vi "Autonomous Independent.vi"   [LabVIEW 2020]
doc: "This VI is called when autonomous begins, and will automatically be terminated when autonomous ends. You can carry out timed or sensor driven robot movement independently without needing to return to the caller."
uses:
  <vilib>/Rock Robotics/Network Tables/NT Read String.vi
  Robot Global Data.vi
panel:
  # "Be sure to right-click and choose Data Operations>>Make Current Value default if you want to save the array values with the VI"
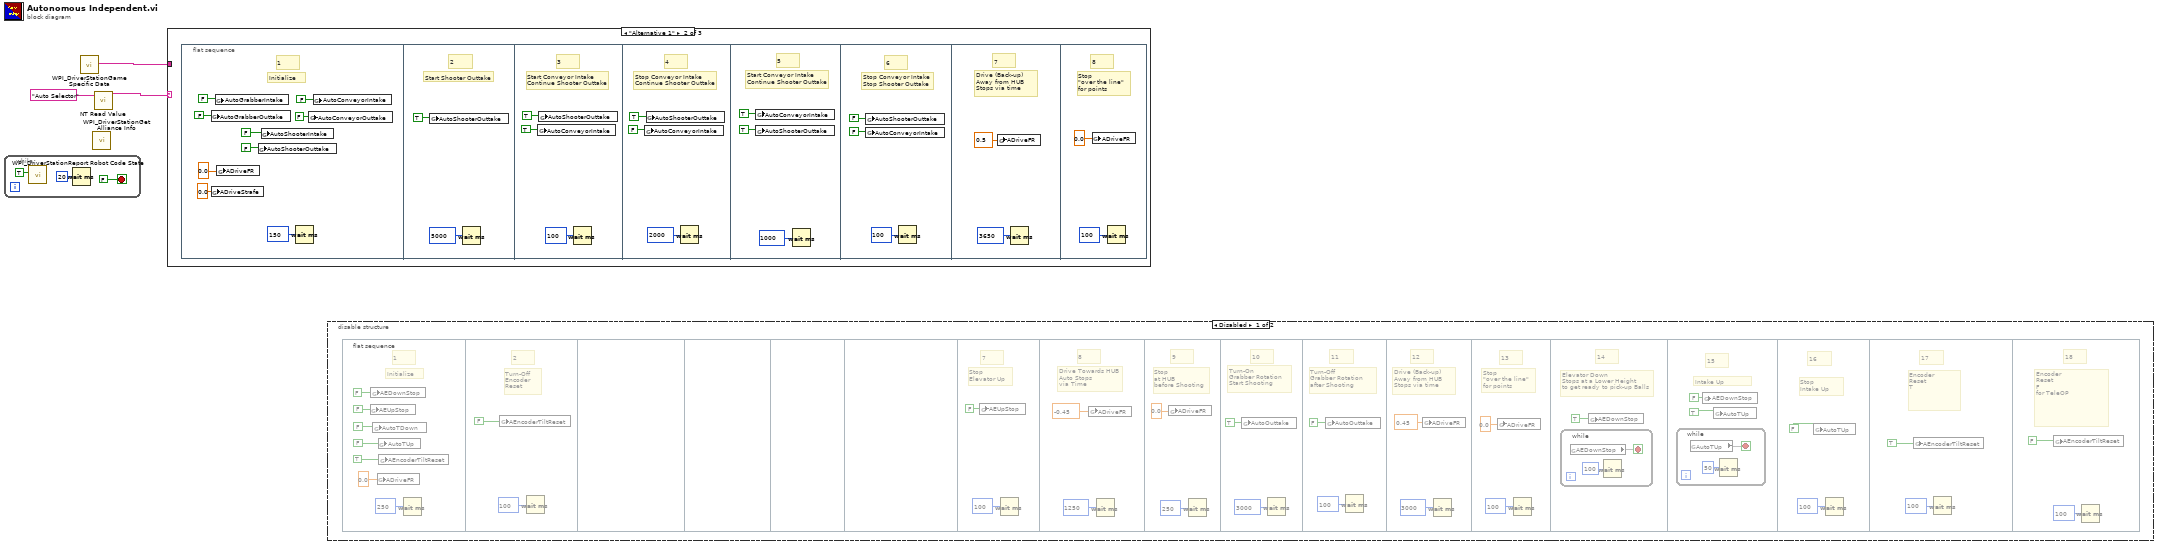
[diagram p0: block diagram]
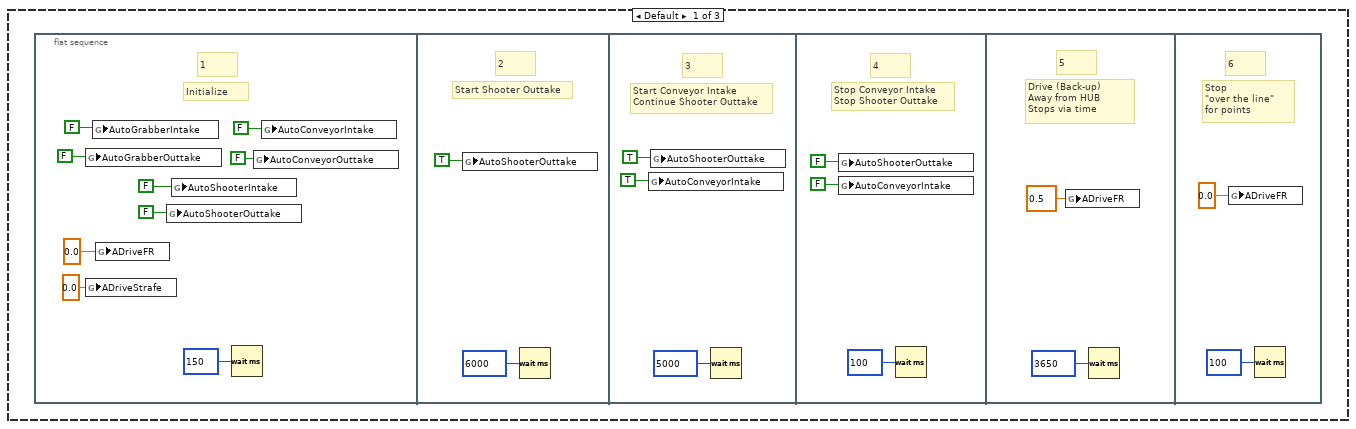
[diagram p3: hidden frame]
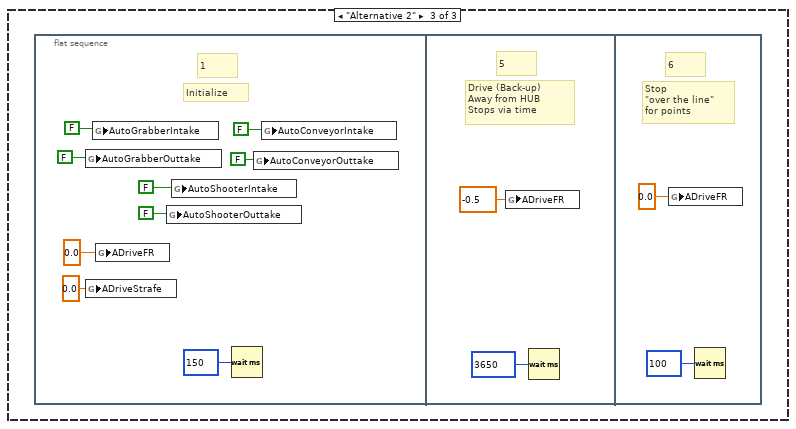
[diagram p4: hidden frame]
diagram:
  n1 = while {
    stop <- FALSE stop-if-true
    n2 = call <vilib>:"WPI_DriverStationReport Robot Code State.vi"("Autonomous"=TRUE) -> ()  [unwired: 10 in, 1 out]
    n3 = Wait (ms)(milliseconds to wait=u32 20) -> ()  [unwired: 1 out]
  }
  n4 = call <vilib>:"WPI_DriverStationGame Specific Data.vi"() -> ("Game Specific Data"=w1:string)  [unwired: 11 in]
  n5 = call <vilib>:"WPI_DriverStationGet Alliance Info.vi"() -> ()  [unwired: 12 out]
  n6 = call-poly <vilib>:"NT Read Value.vi"("Name"="Auto Selector") -> ("String"=w2:string)  [unwired: 9 in, 1 out]
  n7 = case shown="\"Alternative 1\"" w2 {
    tunnel: w1 -> [_ _ _]
    frame Default {
      n8 = flat-sequence {
        frame #0 {
          # "1"
          # "Initialize"
          n9 = global write "Robot Global Data.vi" "AutoGrabberOuttake"(FALSE) -> ()
          n10 = global write "Robot Global Data.vi" "ADriveStrafe"(0.0 ("ADriveFR")) -> ()
          n11 = global write "Robot Global Data.vi" "AutoGrabberIntake"(FALSE) -> ()
          n12 = global write "Robot Global Data.vi" "ADriveFR"(0.0 ("ADriveFR")) -> ()
          n13 = global write "Robot Global Data.vi" "AutoShooterOuttake"(FALSE) -> ()
          n14 = global write "Robot Global Data.vi" "AutoShooterIntake"(FALSE) -> ()
          n15 = Wait (ms)(milliseconds to wait=u32 150) -> ()  [unwired: 1 out]
          n16 = global write "Robot Global Data.vi" "AutoConveyorOuttake"(FALSE) -> ()
          n17 = global write "Robot Global Data.vi" "AutoConveyorIntake"(FALSE) -> ()
        }
        frame #1 {
          # "2"
          # "Start Shooter Outtake"
          n18 = global write "Robot Global Data.vi" "AutoShooterOuttake"(TRUE) -> ()
          n19 = Wait (ms)(milliseconds to wait=u32 6000) -> ()  [unwired: 1 out]
        }
        frame #2 {
          # "Start Conveyor Intake\nContinue Shooter Outtake"
          # "3"
          n20 = global write "Robot Global Data.vi" "AutoConveyorIntake"(TRUE) -> ()
          n21 = global write "Robot Global Data.vi" "AutoShooterOuttake"(TRUE) -> ()
          n22 = Wait (ms)(milliseconds to wait=u32 5000) -> ()  [unwired: 1 out]
        }
        frame #3 {
          # "4"
          # "Stop Conveyor Intake\nStop Shooter Outtake"
          n23 = global write "Robot Global Data.vi" "AutoShooterOuttake"(FALSE) -> ()
          n24 = global write "Robot Global Data.vi" "AutoConveyorIntake"(FALSE) -> ()
          n25 = Wait (ms)(milliseconds to wait=u32 100) -> ()  [unwired: 1 out]
        }
        frame #4 {
          # "5"
          # "Drive (Back-up)\nAway from HUB\nStops via time"
          n26 = global write "Robot Global Data.vi" "ADriveFR"(0.5 ("ADriveFR")) -> ()
          n27 = Wait (ms)(milliseconds to wait=u32 3650) -> ()  [unwired: 1 out]
        }
        frame #5 {
          # "6"
          # "Stop\n\"over the line\"\nfor points"
          n28 = global write "Robot Global Data.vi" "ADriveFR"(0.0 ("ADriveFR")) -> ()
          n29 = Wait (ms)(milliseconds to wait=u32 100) -> ()  [unwired: 1 out]
        }
      }
    }
    frame "Alternative 1" {
      n30 = flat-sequence {
        frame #0 {
          # "1"
          # "Initialize"
          n31 = global write "Robot Global Data.vi" "AutoGrabberOuttake"(FALSE) -> ()
          n32 = global write "Robot Global Data.vi" "ADriveStrafe"(0.0 ("ADriveFR")) -> ()
          n33 = global write "Robot Global Data.vi" "AutoGrabberIntake"(FALSE) -> ()
          n34 = global write "Robot Global Data.vi" "ADriveFR"(0.0 ("ADriveFR")) -> ()
          n35 = global write "Robot Global Data.vi" "AutoShooterOuttake"(FALSE) -> ()
          n36 = global write "Robot Global Data.vi" "AutoShooterIntake"(FALSE) -> ()
          n37 = Wait (ms)(milliseconds to wait=u32 150) -> ()  [unwired: 1 out]
          n38 = global write "Robot Global Data.vi" "AutoConveyorOuttake"(FALSE) -> ()
          n39 = global write "Robot Global Data.vi" "AutoConveyorIntake"(FALSE) -> ()
        }
        frame #1 {
          # "2"
          # "Start Shooter Outtake"
          n40 = global write "Robot Global Data.vi" "AutoShooterOuttake"(TRUE) -> ()
          n41 = Wait (ms)(milliseconds to wait=u32 5000) -> ()  [unwired: 1 out]
        }
        frame #2 {
          # "Start Conveyor Intake\nContinue Shooter Outtake"
          # "3"
          n42 = global write "Robot Global Data.vi" "AutoConveyorIntake"(TRUE) -> ()
          n43 = global write "Robot Global Data.vi" "AutoShooterOuttake"(TRUE) -> ()
          n44 = Wait (ms)(milliseconds to wait=u32 100) -> ()  [unwired: 1 out]
        }
        frame #3 {
          # "Stop Conveyor Intake\nContinue Shooter Outtake"
          # "4"
          n45 = global write "Robot Global Data.vi" "AutoConveyorIntake"(FALSE) -> ()
          n46 = global write "Robot Global Data.vi" "AutoShooterOuttake"(TRUE) -> ()
          n47 = Wait (ms)(milliseconds to wait=u32 2000) -> ()  [unwired: 1 out]
        }
        frame #4 {
          # "Start Conveyor Intake\nContinue Shooter Outtake"
          # "5"
          n48 = global write "Robot Global Data.vi" "AutoConveyorIntake"(TRUE) -> ()
          n49 = global write "Robot Global Data.vi" "AutoShooterOuttake"(TRUE) -> ()
          n50 = Wait (ms)(milliseconds to wait=u32 1000) -> ()  [unwired: 1 out]
        }
        frame #5 {
          # "6"
          # "Stop Conveyor Intake\nStop Shooter Outtake"
          n51 = global write "Robot Global Data.vi" "AutoShooterOuttake"(FALSE) -> ()
          n52 = global write "Robot Global Data.vi" "AutoConveyorIntake"(FALSE) -> ()
          n53 = Wait (ms)(milliseconds to wait=u32 100) -> ()  [unwired: 1 out]
        }
        frame #6 {
          # "7"
          # "Drive (Back-up)\nAway from HUB\nStops via time"
          n54 = global write "Robot Global Data.vi" "ADriveFR"(0.5 ("ADriveFR")) -> ()
          n55 = Wait (ms)(milliseconds to wait=u32 3650) -> ()  [unwired: 1 out]
        }
        frame #7 {
          # "8"
          # "Stop\n\"over the line\"\nfor points"
          n56 = global write "Robot Global Data.vi" "ADriveFR"(0.0 ("ADriveFR")) -> ()
          n57 = Wait (ms)(milliseconds to wait=u32 100) -> ()  [unwired: 1 out]
        }
      }
    }
    frame "Alternative 2" {
      n58 = flat-sequence {
        frame #0 {
          # "1"
          # "Initialize"
          n59 = global write "Robot Global Data.vi" "AutoGrabberOuttake"(FALSE) -> ()
          n60 = global write "Robot Global Data.vi" "ADriveStrafe"(0.0 ("ADriveFR")) -> ()
          n61 = global write "Robot Global Data.vi" "AutoGrabberIntake"(FALSE) -> ()
          n62 = global write "Robot Global Data.vi" "ADriveFR"(0.0 ("ADriveFR")) -> ()
          n63 = global write "Robot Global Data.vi" "AutoShooterOuttake"(FALSE) -> ()
          n64 = global write "Robot Global Data.vi" "AutoShooterIntake"(FALSE) -> ()
          n65 = Wait (ms)(milliseconds to wait=u32 150) -> ()  [unwired: 1 out]
          n66 = global write "Robot Global Data.vi" "AutoConveyorOuttake"(FALSE) -> ()
          n67 = global write "Robot Global Data.vi" "AutoConveyorIntake"(FALSE) -> ()
        }
        frame #1 {
          # "5"
          # "Drive (Back-up)\nAway from HUB\nStops via time"
          n68 = global write "Robot Global Data.vi" "ADriveFR"(-0.5 ("ADriveFR")) -> ()
          n69 = Wait (ms)(milliseconds to wait=u32 3650) -> ()  [unwired: 1 out]
        }
        frame #2 {
          # "6"
          # "Stop\n\"over the line\"\nfor points"
          n70 = global write "Robot Global Data.vi" "ADriveFR"(0.0 ("ADriveFR")) -> ()
          n71 = Wait (ms)(milliseconds to wait=u32 100) -> ()  [unwired: 1 out]
        }
      }
    }
  }
  n72 = disable-structure shown="Disabled" {
    frame Disabled {
      n73 = flat-sequence {
        frame #0 {
          # "1"
          # "Initialize"
          n74 = global write "Robot Global Data.vi" "AEUpStop"(FALSE) -> ()
          n75 = global write "Robot Global Data.vi" "AEDownStop"(FALSE) -> ()
          n76 = global write "Robot Global Data.vi" "AutoTDown"(FALSE) -> ()
          n77 = global write "Robot Global Data.vi" "ADriveFR"(0.0 ("ADriveFR")) -> ()
          n78 = global write "Robot Global Data.vi" "AutoTUp"(FALSE) -> ()
          n79 = global write "Robot Global Data.vi" "AEncoderTiltReset"(TRUE) -> ()
          n80 = Wait (ms)(milliseconds to wait=u32 250) -> ()  [unwired: 1 out]
        }
        frame #1 {
          # "2"
          # "Turn-Off\nEncoder\nReset"
          n81 = global write "Robot Global Data.vi" "AEncoderTiltReset"(FALSE) -> ()
          n82 = Wait (ms)(milliseconds to wait=u32 100) -> ()  [unwired: 1 out]
        }
        frame #2 {
        }
        frame #3 {
        }
        frame #4 {
        }
        frame #5 {
        }
        frame #6 {
          # "7"
          # "Stop\nElevator Up"
          n83 = global write "Robot Global Data.vi" "AEUpStop"(FALSE) -> ()
          n84 = Wait (ms)(milliseconds to wait=u32 100) -> ()  [unwired: 1 out]
        }
        frame #7 {
          # "8"
          # "Drive Towards HUB\nAuto Stops\nvia Time"
          n85 = global write "Robot Global Data.vi" "ADriveFR"(-0.45 ("ADriveFR")) -> ()
          n86 = Wait (ms)(milliseconds to wait=u32 1250) -> ()  [unwired: 1 out]
        }
        frame #8 {
          # "9"
          # "Stop\nat HUB\nbefore Shooting"
          n87 = global write "Robot Global Data.vi" "ADriveFR"(0.0 ("ADriveFR")) -> ()
          n88 = Wait (ms)(milliseconds to wait=u32 250) -> ()  [unwired: 1 out]
        }
        frame #9 {
          # "10"
          # "Turn-On\nGrabber Rotation\nStart Shooting"
          n89 = global write "Robot Global Data.vi" "AutoOuttake"(TRUE ("AutoOuttake")) -> ()
          n90 = Wait (ms)(milliseconds to wait=u32 3000) -> ()  [unwired: 1 out]
        }
        frame #10 {
          # "11"
          # "Turn-Off\nGrabber Rotation\nafter Shooting"
          n91 = global write "Robot Global Data.vi" "AutoOuttake"(FALSE ("AutoOuttake")) -> ()
          n92 = Wait (ms)(milliseconds to wait=u32 100) -> ()  [unwired: 1 out]
        }
        frame #11 {
          # "12"
          # "Drive (Back-up)\nAway from HUB\nStops via time"
          n93 = global write "Robot Global Data.vi" "ADriveFR"(0.45 ("ADriveFR")) -> ()
          n94 = Wait (ms)(milliseconds to wait=u32 3000) -> ()  [unwired: 1 out]
        }
        frame #12 {
          # "13"
          # "Stop\n\"over the line\"\nfor points"
          n95 = global write "Robot Global Data.vi" "ADriveFR"(0.0 ("ADriveFR")) -> ()
          n96 = Wait (ms)(milliseconds to wait=u32 100) -> ()  [unwired: 1 out]
        }
        frame #13 {
          # "14"
          # "Elevator Down\nStops at a Lower Height\nto get ready to pick-up Balls"
          n97 = while {
            stop <- w92 stop-if-true
            n98 = global read "Robot Global Data.vi" "AEDownStop"() -> (w92)
            n99 = Wait (ms)(milliseconds to wait=u32 100) -> ()  [unwired: 1 out]
          }
          n100 = global write "Robot Global Data.vi" "AEDownStop"(TRUE) -> ()
        }
        frame #14 {
          # "Intake Up"
          # "15"
          n101 = while {
            stop <- w96 stop-if-true
            n102 = global read "Robot Global Data.vi" "AutoTUp"() -> (w96)
            n103 = Wait (ms)(milliseconds to wait=u32 50) -> ()  [unwired: 1 out]
          }
          n104 = global write "Robot Global Data.vi" "AEDownStop"(FALSE) -> ()
          n105 = global write "Robot Global Data.vi" "AutoTUp"(TRUE) -> ()
        }
        frame #15 {
          # "Stop\nIntake Up"
          # "16"
          n106 = global write "Robot Global Data.vi" "AutoTUp"(FALSE) -> ()
          n107 = Wait (ms)(milliseconds to wait=u32 100) -> ()  [unwired: 1 out]
        }
        frame #16 {
          # "17"
          # "Encoder\nReset\nT"
          n108 = global write "Robot Global Data.vi" "AEncoderTiltReset"(TRUE) -> ()
          n109 = Wait (ms)(milliseconds to wait=u32 100) -> ()  [unwired: 1 out]
        }
        frame #17 {
          # "18"
          # "Encoder\nReset\nF \nfor TeleOP"
          n110 = global write "Robot Global Data.vi" "AEncoderTiltReset"(FALSE) -> ()
          n111 = Wait (ms)(milliseconds to wait=u32 100) -> ()  [unwired: 1 out]
        }
      }
    }
    frame Enabled {
    }
  }
